vi "perform.vi"(8 "error in (no error)":errorcluster, 10 "Sensor Data":T2 {"Robot Heading" format="%05.1f"; "Wind Direction" format="%05.1f"}, 11 "Mission in":refnum<class "Mission.lvclass">) -> (0 "error out":errorcluster, 2 "Desired Location":T1, 3 "Mission out":refnum<class "Mission.lvclass">)   [LabVIEW 2011, in "Mission.lvclass"]
doc: "Guide the mission by providing the current desired location. Sensor data is supplied to allow the mission to keep track of its mission progress internally."
uses:
  Mission.lvclass
  2-RIO/2 Typedefs/sensorData.ctl
  2-RIO/2 Typedefs/UTM Location.ctl
  2-RIO/2 Typedefs/heading.ctl
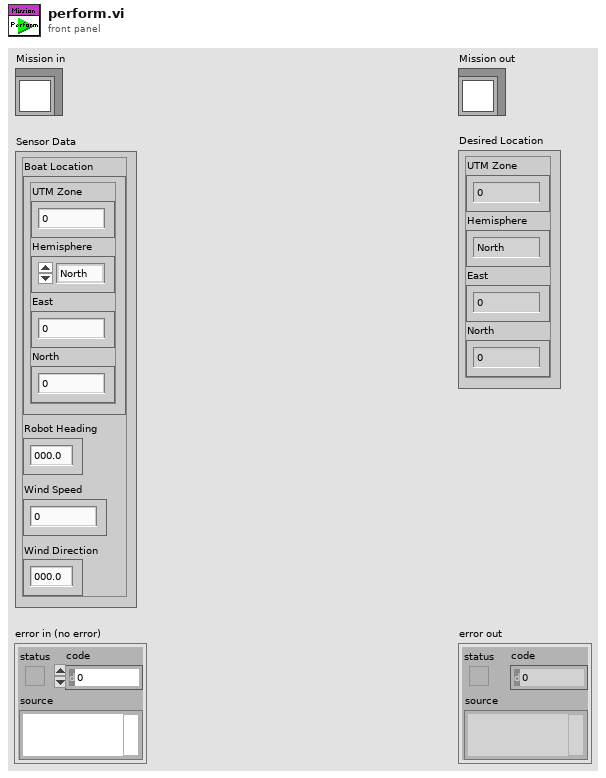
[diagram p1: front panel]
types:
  T1 = typedef "UTM Location.ctl" = cluster{"UTM Zone":dbl, "Hemisphere":enum16{"North", "South"}, "East":dbl, "North":dbl}
  T2 = typedef "sensorData.ctl" = cluster{"Boat Location":T1, "Robot Heading ":T3, "Wind Speed":dbl, "Wind Direction":T3}
  T3 = typedef "heading.ctl" = dbl
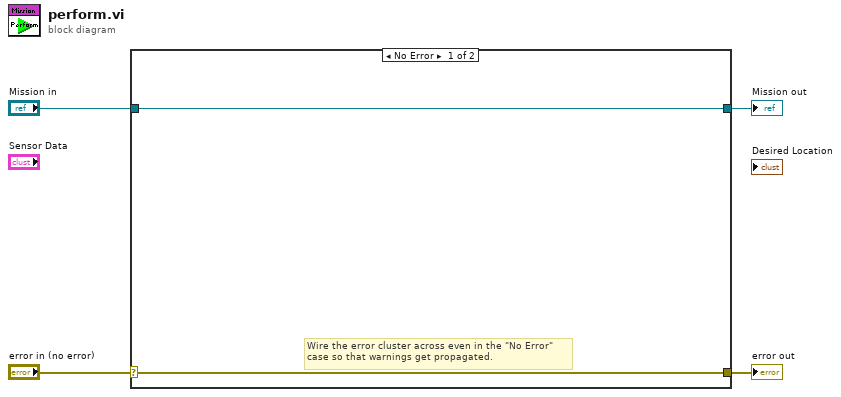
[diagram p0: block diagram]
diagram:
  n1 = case shown="No Error" "error in (no error)" {
    selector: "error in (no error)" -> [w5 w8]
    tunnel: [w5 w8] -> w3
    tunnel: [w6 w7] -> w1
    tunnel: "Mission in" -> [w6 w7]
    frame No Error {
      # "Wire the error cluster across even in the \"No Error\"\ncase so that warnings get propagated."
    }
    frame Error {
    }
  }
  "error out" <- w3
  "Mission out" <- w1
